vi "GeneratePiezoLaserWaveform.vi"(7 "Acquition Time (sec)":dbl, 8 "error out":errorcluster, 9 "Start or Continue?":bool, 10 "Piezo Mode":string, 11 "Laser Mode":string) -> (0 "error out":errorcluster, 1 "Number of Samples":i32, 2 "Waveforms":waveform(dbl)[](array[waveform]))   [LabVIEW 2015]
uses:
  NIDAQControls/NIDAQGlobals.vi
  NIDAQControls/StateGlobals.vi
  Andor/LiveImage_Global.vi
panel:
  out "Waveform Graph":waveform(dbl)[](graph)
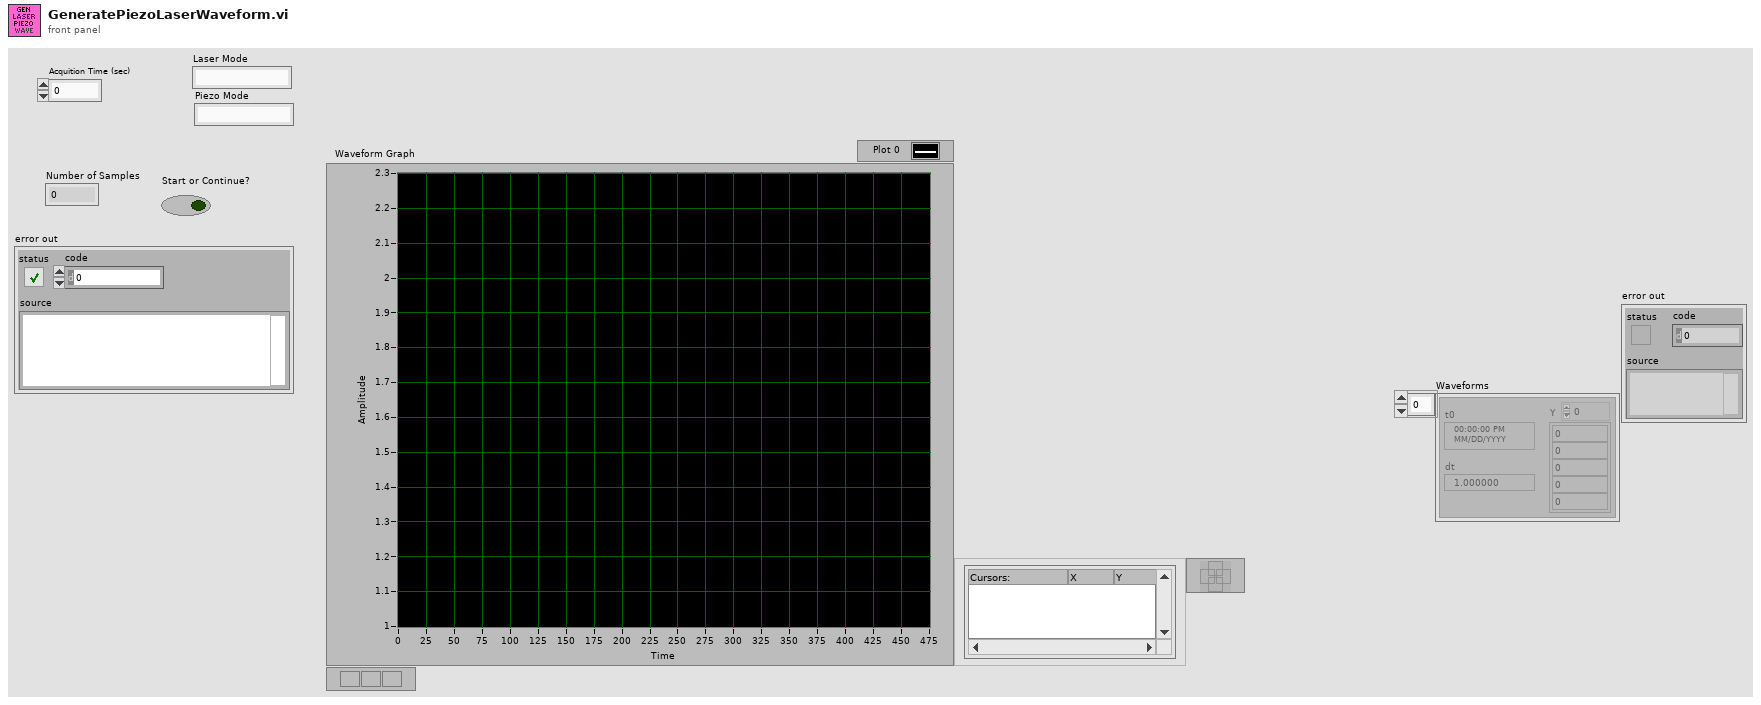
[diagram p1: front panel]
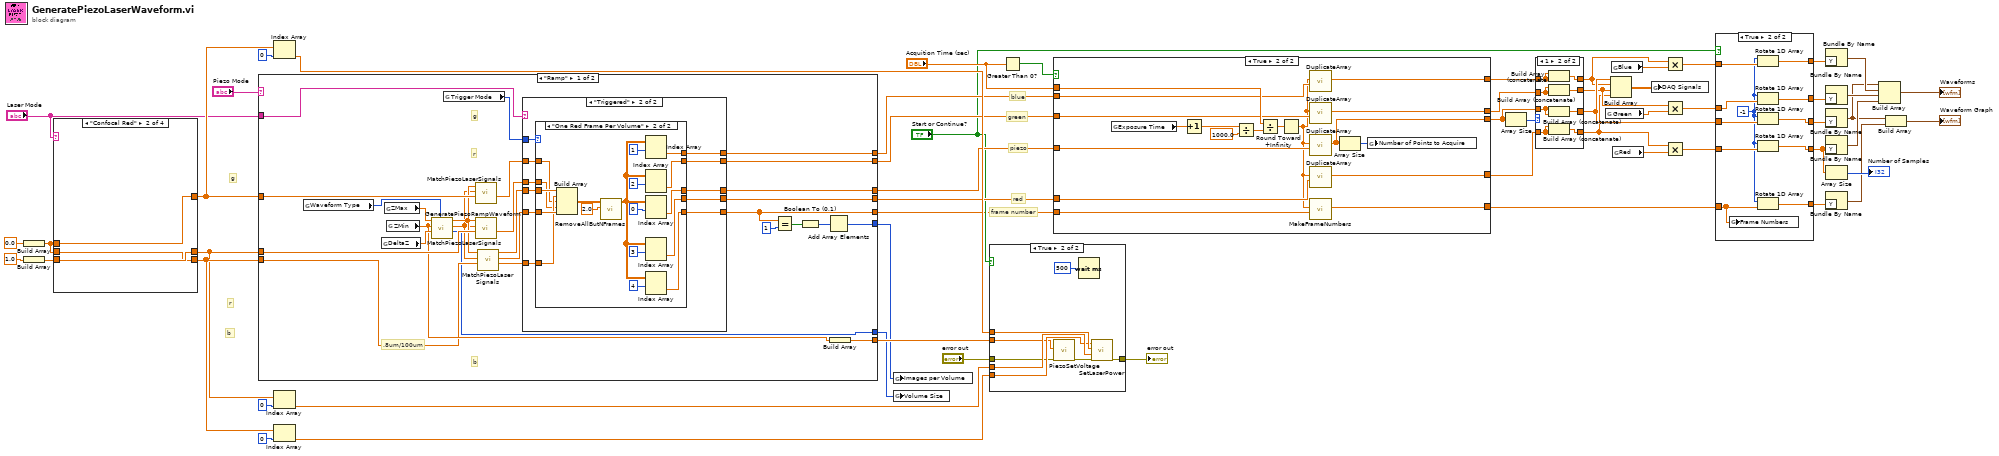
[diagram p0: block diagram]
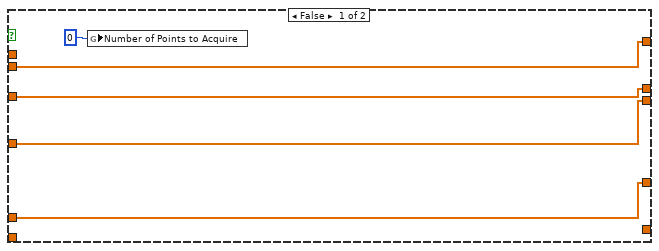
[diagram p4: hidden frame]
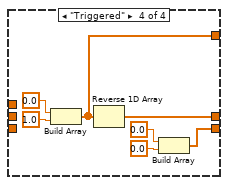
[diagram p8: hidden frame]
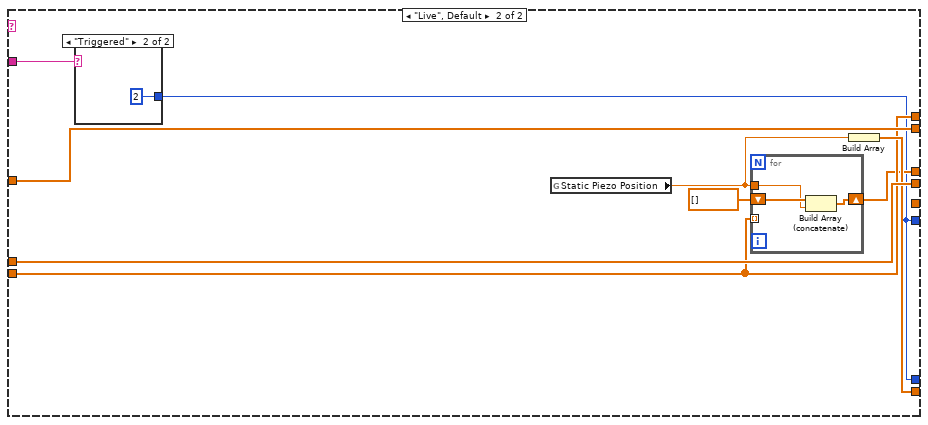
[diagram p11: hidden frame]
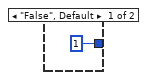
[diagram p12: hidden frame]
diagram:
  # "b"
  # "r"
  # "g"
  # "blue"
  # "piezo"
  # "red"
  # "green"
  # "frame number"
  n1 = Build Array(0.0 ("element")) -> (w20:dbl[])
  n2 = Build Array(1.0 ("element")) -> (w22:dbl[])
  n3 = case shown="\"Confocal Red\"" "Laser Mode" {
    tunnel: [w60 w63 w67 w69] -> w51
    tunnel: [w59 w62 w65 w70] -> w52
    tunnel: [w61 w64 w66 w68] -> w2
    tunnel: w20 -> [w61 w63 w66 _]
    tunnel: w22 -> [w60 w64 w65 _]
    tunnel: w20 -> [w59 w62 w67 _]
    frame "Confocal Green" {
    }
    frame "Confocal Red" {
    }
    frame "Confocal Blue", Default {
    }
    frame "Triggered" {
      n4 = Build Array(0.0 ("element"), 1.0 ("element")) -> (w69:dbl[])
      n5 = Reverse 1D Array(array=w69) -> (reversed array=w68:dbl[])
      n6 = Build Array(0.0 ("element"), 0.0 ("element")) -> (w70:dbl[])
    }
  }
  n7 = case shown="\"Ramp\"" "Piezo Mode" {
    tunnel: [w86 w144] -> w31
    tunnel: w52 -> [w94 w145]
    tunnel: w51 -> [w100 w148]
    tunnel: w2 -> [w101 w149]
    tunnel: [w79 w149] -> w30
    tunnel: [w81 w148] -> w28
    tunnel: [w83 w145] -> w29
    tunnel: [w99 w147] -> w26
    tunnel: [w75 _] -> w10
    tunnel: [w92 w141] -> w4
    tunnel: [w87 w141] -> w3
    tunnel: "Laser Mode" -> [w76 w142]
    frame "Ramp" {
      # "g"
      # "r"
      # "b"
      # ".8um/100um"
      n8 = global read "NIDAQGlobals.vi" "Waveform Type"() -> (w91:enum16{"Triangle", "Sawtooth"})
      n9 = global read "NIDAQGlobals.vi" "DeltaZ"() -> (w98:dbl)
      n10 = global read "NIDAQGlobals.vi" "ZMax"() -> (w96:dbl)
      n11 = global read "NIDAQGlobals.vi" "ZMin"() -> (w97:dbl)
      n12 = call "GeneratePiezoRampWaveform.vi"("Waveform Type"=w91, "Delta"=w98, "Min"=w97, "Max"=w96) -> ("Volume Size"=w92:i32, "Volume Number"=w93:dbl[], "Ramp"=w95:dbl[])  [unwired: 5 in]
      n13 = global read "NIDAQGlobals.vi" "Trigger Mode"() -> (w78:enum16{"Normal", "One Red Frame Per Volume"})
      n14 = call "MatchPiezoLaserSignals.vi"("LaserSigIn"=w100, "VolumeNumberIn"=w93, "PiezoSig"=w95) -> ("LaserSigOut"=w82:dbl[])  [unwired: 5 in, 2 out]
      n15 = call "MatchPiezoLaserSignals.vi"("LaserSigIn"=w101, "VolumeNumberIn"=w93, "PiezoSig"=w95) -> ("LaserSigOut"=w80:dbl[])  [unwired: 5 in, 2 out]
      n16 = call "MatchPiezoLaserSignals.vi"("LaserSigIn"=w94, "VolumeNumberIn"=w93, "PiezoSig"=w95) -> ("LaserSigOut"=w84:dbl[], "VolumeNumberOut"=w85:dbl[], "PiezoSigOut"=w77:dbl[])  [unwired: 5 in]
      n17 = case shown="\"Triggered\"" w76 {
        tunnel: [w103 w117] -> w86
        tunnel: w85 -> [w102 w116]
        tunnel: [w102 w115] -> w75
        tunnel: w84 -> [w104 w114]
        tunnel: [w104 w113] -> w83
        tunnel: w82 -> [w106 w112]
        tunnel: [w106 w111] -> w81
        tunnel: w80 -> [w105 w110]
        tunnel: [w105 w109] -> w79
        tunnel: w78 -> [_ w108]
        tunnel: w77 -> [w103 w107]
        frame "False", Default {
        }
        frame "Triggered" {
          n18 = case shown="\"One Red Frame Per Volume\"" w108 {
            tunnel: w107 -> [w121 w132]
            tunnel: [w121 w131] -> w117
            tunnel: w116 -> [w120 w130]
            tunnel: [w120 w129] -> w115
            tunnel: w114 -> [w118 w128]
            tunnel: [w118 w127] -> w113
            tunnel: w112 -> [w119 w126]
            tunnel: [w119 w125] -> w111
            tunnel: w110 -> [w122 w124]
            tunnel: [w122 w123] -> w109
            frame "Normal", Default {
            }
            frame "One Red Frame Per Volume" {
              n19 = Build Array(w132, w128, w126, w124, w130) -> (w140:dbl[][])
              n20 = call "RemoveAllButNFrames.vi"("Laser to delete (BGR)"=2.0, "Array"=w140) -> ("Array 2"=w133:dbl[][])  [unwired: 9 in]
              n21 = Index Array(array=w133, index (row)=1) -> (element=w127:dbl[])  [unwired: 1 in]
              n22 = Index Array(array=w133, index (row)=2) -> (element=w125:dbl[])  [unwired: 1 in]
              n23 = Index Array(array=w133, index (row)=0) -> (element=w131:dbl[])  [unwired: 1 in]
              n24 = Index Array(array=w133, index (row)=3) -> (element=w123:dbl[])  [unwired: 1 in]
              n25 = Index Array(array=w133, index (row)=4) -> (element=w129:dbl[])  [unwired: 1 in]
            }
          }
        }
      }
      n26 = Equal?(x=w75, y=1) -> (x = y?=w89:bool[])
      n27 = Boolean To (0,1)(Boolean=w89) -> (0, 1=w88:i16[])
      n28 = Add Array Elements(numeric array=w88) -> (sum=w87:i16)
      n29 = Build Array(w97) -> (w99:dbl[])
    }
    frame "Live", Default {
      n30 = case shown="\"Triggered\"" w142 {
        tunnel: [1 ("Volume Size") 2 ("Volume Size")] -> w141
        frame "False", Default {
        }
        frame "Triggered" {
        }
      }
      n31 = global read "NIDAQGlobals.vi" "Static Piezo Position"() -> (w143:dbl)
      n32 = for {
        tunnel: w145 -> [_] mode=indexing
        tunnel: w143 -> [w152]
        shift-right: [w154] -> w144
        shift-left: dbl[] [] -> [w153]
        n33 = Build Array (concatenate)(w153, w152) -> (w154:dbl[])
      }
      n34 = Build Array(w143) -> (w147:dbl[])
    }
  }
  n35 = Index Array(array=w51, index=0) -> (element=w54:dbl)
  n36 = Index Array(array=w2, index=0) -> (element=w55:dbl)
  n37 = Index Array(array=w52, index=0) -> (element=w53:dbl)
  n38 = global write "NIDAQGlobals.vi" "Images per Volume"(w3) -> ()
  n39 = global write "NIDAQGlobals.vi" "Volume Size"(w4) -> ()
  n40 = case shown="True" "Start or Continue?" {
    tunnel: w55 -> [_ w163]
    tunnel: w54 -> [_ w162]
    tunnel: w53 -> [_ w161]
    tunnel: [w155 w160] -> w36
    tunnel: w26 -> [_ w159]
    tunnel: "error out" -> [w155 w158]
    frame False {
    }
    frame True {
      n41 = call "PiezoSetVoltage.vi"("error in"=w158, "data"=w159) -> ("error out"=w157:errorcluster)  [unwired: 9 in]
      n42 = Wait (ms)(milliseconds to wait=u32 500) -> ()  [unwired: 1 out]
      n43 = call "SetLaserPower.vi"("error in"=w157, "AOTF3"=w163, "AOTF2"=w162, "AOTF1"=w161) -> ("error out"=w160:errorcluster)  [unwired: 7 in]
    }
  }
  "error out" <- w36
  n44 = Greater Than 0?(x="Acquition Time (sec)") -> (x > 0?=w32:bool)
  n45 = case shown="True" w32 {
    tunnel: w31 -> [w168 w176]
    tunnel: [w168 w173] -> w12
    tunnel: [w167 w174] -> w14
    tunnel: w30 -> [w167 w175]
    tunnel: w29 -> [w166 w177]
    tunnel: [w166 w179] -> w18
    tunnel: w28 -> [w165 w178]
    tunnel: [w165 w180] -> w16
    tunnel: "Acquition Time (sec)" -> [_ w183]
    tunnel: w10 -> [_ w171]
    tunnel: [_ w169] -> w9
    frame False {
      n46 = global write "StateGlobals.vi" "Number of Points to Acquire"(0 ("Number of Points to Acquire")) -> ()
    }
    frame True {
      n47 = global read "LiveImage_Global.vi" "Exposure Time"() -> (w186:dbl)
      n48 = Increment(x=w186) -> (x+1=w185:dbl)
      n49 = Divide(x=w185, y=1000.0) -> (x/y=w182:dbl)
      n50 = Divide(x=w183, y=w182) -> (x/y=w181:dbl)
      n51 = Round Toward +Infinity(x=w181) -> (ceil(x): smallest int >= x=w170:dbl)
      n52 = call "DuplicateArray.vi"("Array"=w177, "Number of frames"=w170) -> ("Duplicated Array"=w179:dbl[])  [unwired: 9 in]
      n53 = call "DuplicateArray.vi"("Array"=w178, "Number of frames"=w170) -> ("Duplicated Array"=w180:dbl[])  [unwired: 9 in]
      n54 = call "DuplicateArray.vi"("Array"=w176, "Number of frames"=w170) -> ("Duplicated Array"=w173:dbl[])  [unwired: 9 in]
      n55 = call "DuplicateArray.vi"("Array"=w175, "Number of frames"=w170) -> ("Duplicated Array"=w174:dbl[])  [unwired: 9 in]
      n56 = call "MakeFrameNumbers.vi"("Array"=w171, "Number of frames"=w170) -> ("Frame Number Array"=w169:dbl[])  [unwired: 9 in]
      n57 = Array Size(array=w173) -> (size(s)=w172:i32)
      n58 = global write "StateGlobals.vi" "Number of Points to Acquire"(w172) -> ()
    }
  }
  n59 = Array Size(array=w12) -> (size(s)=w11:i32)
  n60 = case shown="1" w11 {
    tunnel: [w190 w198] -> w19
    tunnel: w12 -> [w190 w197]
    tunnel: [w189 w195] -> w17
    tunnel: w18 -> [w189 w196]
    tunnel: w16 -> [w188 w194]
    tunnel: [w188 w193] -> w15
    tunnel: w14 -> [w187 w192]
    tunnel: [w187 w191] -> w13
    frame 0, Default {
    }
    frame 1 {
      n61 = Build Array (concatenate)(w196, w196) -> (w195:dbl[])
      n62 = Build Array (concatenate)(w194, w194) -> (w193:dbl[])
      n63 = Build Array (concatenate)(w197, w197) -> (w198:dbl[])
      n64 = Build Array (concatenate)(w192, w192) -> (w191:dbl[])
    }
  }
  n65 = global read "NIDAQGlobals.vi" "Green"() -> (w48:dbl)
  n66 = Build Array(w19, w17, w15, w13) -> (w24:dbl[][])
  n67 = global read "NIDAQGlobals.vi" "Blue"() -> (w46:dbl)
  n68 = global read "NIDAQGlobals.vi" "Red"() -> (w50:dbl)
  n69 = global write "NIDAQGlobals.vi" "DAQ Signals"(w24) -> ()
  n70 = Multiply(x=w17, y=w46) -> (x*y=w45:dbl[])
  n71 = Multiply(x=w15, y=w48) -> (x*y=w47:dbl[])
  n72 = Multiply(x=w13, y=w50) -> (x*y=w49:dbl[])
  n73 = case shown="True" "Start or Continue?" {
    tunnel: w49 -> [w199 w213]
    tunnel: w47 -> [w200 w212]
    tunnel: w45 -> [w201 w211]
    tunnel: [w202 w210] -> w44
    tunnel: [w201 w209] -> w43
    tunnel: [w200 w208] -> w42
    tunnel: [w199 w207] -> w34
    tunnel: w19 -> [w202 w206]
    tunnel: w9 -> [_ w203]
    tunnel: [_ w204] -> w8
    frame False {
    }
    frame True {
      w205 = -1 ("n")
      n74 = global write "NIDAQGlobals.vi" "Frame Numbers"(w203) -> ()
      n75 = Rotate 1D Array(1:w211, 2:w205) -> (0:w209:dbl[])
      n76 = Rotate 1D Array(1:w212, 2:w205) -> (0:w208:dbl[])
      n77 = Rotate 1D Array(1:w206, 2:w205) -> (0:w210:dbl[])
      n78 = Rotate 1D Array(1:w213, 2:w205) -> (0:w207:dbl[])
      n79 = Rotate 1D Array(1:w203, 2:w205) -> (0:w204:dbl[])
    }
  }
  n80 = Bundle By Name("Y"=w43) -> (w41:waveform(dbl))  [unwired: 1 in]
  n81 = Bundle By Name("Y"=w42) -> (w40:waveform(dbl))  [unwired: 1 in]
  n82 = Bundle By Name("Y"=w44) -> (w6:waveform(dbl))  [unwired: 1 in]
  n83 = Bundle By Name("Y"=w34) -> (w38:waveform(dbl))  [unwired: 1 in]
  n84 = Array Size(array=w34) -> (size(s)=→"Number of Samples":i32)
  n85 = Bundle By Name("Y"=w8) -> (w7:waveform(dbl))  [unwired: 1 in]
  n86 = Build Array(w6, w41, w40, w38) -> (→"Waveforms":waveform(dbl)[])
  n87 = Build Array(w6, w7) -> (→"Waveform Graph":waveform(dbl)[])
